vi "VRAI_COULEUR.vi"(9 "IMAGE COLORS":i32[](array[numeric]), 11 "CLUT":i32[](array[numeric])) -> (1 "REAL IMAGE COLORS":i32[](array[numeric]), 3 "STRING FOR MATLAB":string[](array[string]))   [LabVIEW 2013]
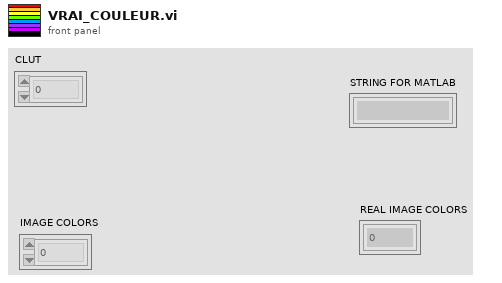
[diagram p1: front panel]
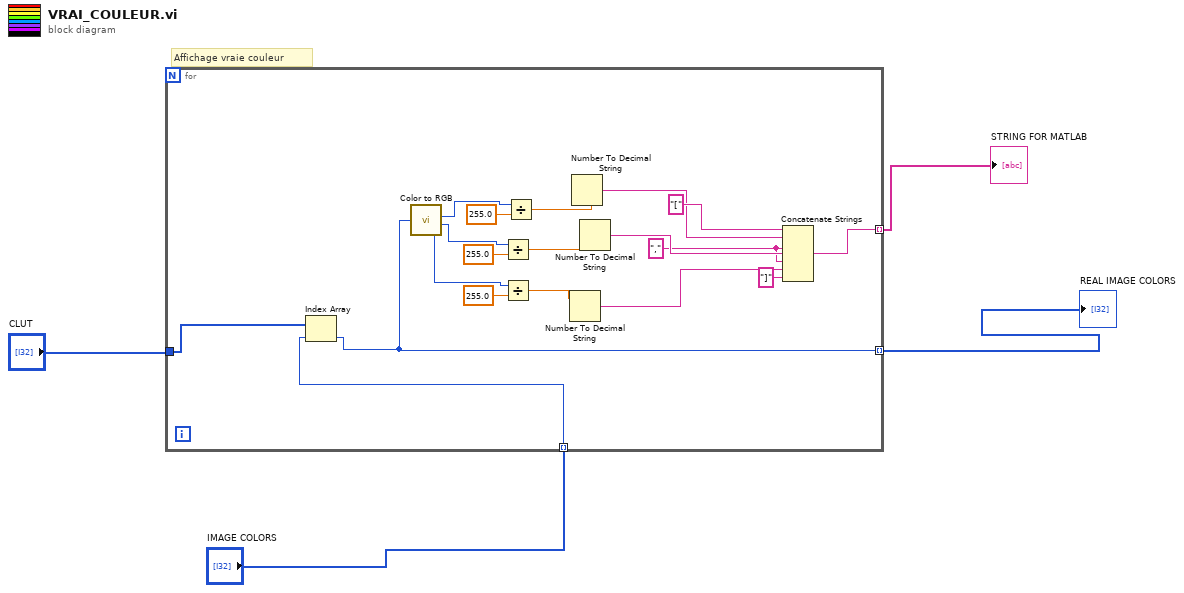
[diagram p0: block diagram]
diagram:
  # "Affichage vraie couleur"
  n1 = for {
    tunnel: "CLUT" -> [w23]
    tunnel: [w21] -> w1 mode=indexing
    tunnel: "IMAGE COLORS" -> [w22] mode=indexing
    tunnel: [w5] -> w2 mode=indexing
    w8 = "," ("string")
    n2 = Index Array(array=w23, index=w22) -> (element=w21:i32)
    n3 = call <vilib>:"Color to RGB.vi"("Color"=w21) -> ("R"=w17:u8, "G"=w16:u8, "B"=w15:u8)  [unwired: 1 out]
    n4 = Divide(x=w16, y=255.0) -> (x/y=w13:dbl)
    n5 = Divide(x=w15, y=255.0) -> (x/y=w14:dbl)
    n6 = Divide(x=w17, y=255.0) -> (x/y=w12:dbl)
    n7 = Number To Decimal String(number=w14) -> (decimal integer string=w7:string)  [unwired: 1 in]
    n8 = Number To Decimal String(number=w12) -> (decimal integer string=w10:string)  [unwired: 1 in]
    n9 = Number To Decimal String(number=w13) -> (decimal integer string=w9:string)  [unwired: 1 in]
    n10 = Concatenate Strings("[" ("string"), w10, w8, w9, w8, w7, "]" ("string")) -> (w5:string)
  }
  "REAL IMAGE COLORS" <- w1
  "STRING FOR MATLAB" <- w2
